vi "Tosca-Splash Screen.vi"(7 "Splash":bool) -> (4 "VI ref":refnum<vi>)   [LabVIEW 2020]
uses:
  Tosca-Globals.vi
  <resource>/objmgr/daqmx.rc
panel:
  out "Loading":string
  in  "OK Button":bool
  out "Version":string
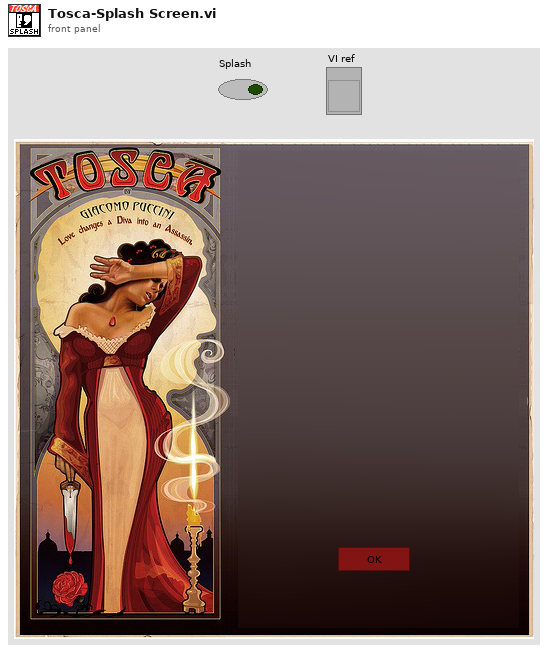
[diagram p1: front panel]
types:
  T1 = cluster{"Major":i32, "Minor":i32, "Build":i32, "Private":i32, "FileVersion":string, "ProductName":string, "InternalName":string, "CompanyName":string, "LegalCopyright":string, "FileDescription":string}
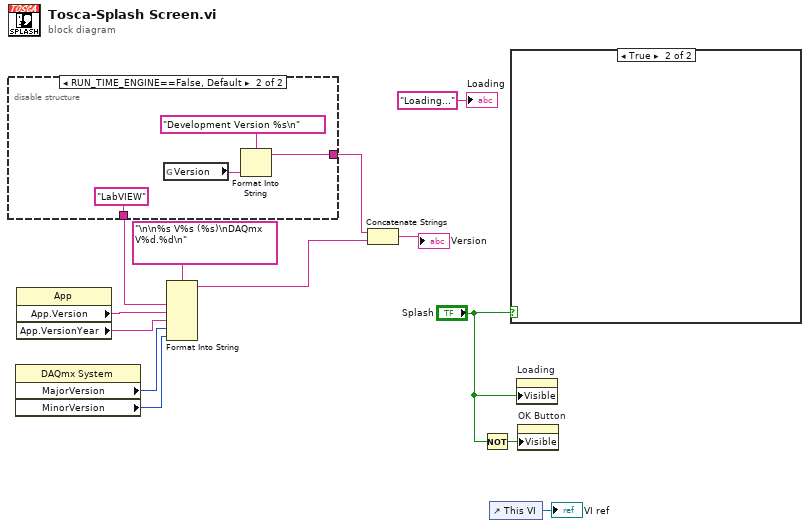
[diagram p0: block diagram]
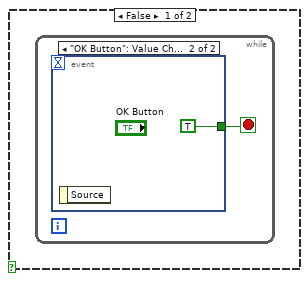
[diagram p2: hidden frame]
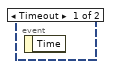
[diagram p3: hidden frame]
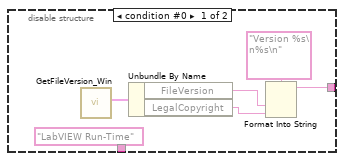
[diagram p4: hidden frame]
diagram:
  n1 = disable-structure shown="RUN_TIME_ENGINE==False, Default" {
    disable-tunnel: [w17 w22] -> w10
    disable-tunnel: ["LabVIEW Run-Time" "LabVIEW"] -> w13
    frame condition #0 {
      n2 = call "GetFileVersion_Win.vi"() -> ("File Info Out"=w18:T1)  [unwired: 9 in, 2 out]
      n3 = Unbundle By Name(w18) -> ("FileVersion"=w16:string, "LegalCopyright"=w15:string)
      n4 = Format Into String(format string="Version %s\n%s\n", w16, w15) -> (resulting string=w17:string)  [unwired: 2 in, 1 out]
    }
    frame condition #1 (active) {
      n5 = global read "Tosca-Globals.vi" "Version"() -> (w20:string)
      n6 = Format Into String(format string="Development Version %s\n" ("PF Version"), w20) -> (resulting string=w22:string)  [unwired: 2 in, 1 out]
    }
  }
  n7 = property class="DAQmx System"() -> ("MajorVersion"=w6:u32, "MinorVersion"=w5:u32)  [unwired: 2 in, 2 out]
  n8 = property class="App"() -> ("App.Version"=w8:string, "App.VersionYear"=w7:string)  [unwired: 2 in, 2 out]
  n9 = Format Into String(format string="\n\n%s V%s (%s)\nDAQmx V%d.%d\n", w13, w8, w7, w6, w5) -> (resulting string=w11:string)  [unwired: 2 in, 1 out]
  n10 = Concatenate Strings(w10, w11) -> (→"Version":string)
  n11 = Not(x="Splash") -> (.not. x?=w4:bool)
  n12 = control-ref of="This VI"() -> (→"VI ref":refnum<vi>)
  n13 = case shown="True" "Splash" {
    frame False {
      n14 = while {
        stop <- w24 stop-if-true
        n15 = event shown="[1] \"OK Button\": Value Change" {
          selector: _ -> [_ _]
          dyn-events: _ -> [_ _]
          timeout: _ -> [_ _]
          tunnel: [_ TRUE] -> w24
          event Timeout {
            n16 = event-data() -> ()  [unwired: 1 in, 1 out]
          }
          event "OK Button": Value Change {
            n17 = event-data() -> ()  [unwired: 1 in, 1 out]
          }
        }
      }
    }
    frame True {
    }
  }
  n18 = property on="Loading" class="Str"("Visible"="Splash") -> ()  [unwired: 2 in, 2 out]
  n19 = property on="OK Button" class="Bool"("Visible"=w4) -> ()  [unwired: 2 in, 2 out]
  "Loading" <- "Loading..." ("Loading")
